vi "Compute Centroid.vi"(0 "Pixel0":bool, 1 "Image Width":u16, 4 "Image Height":u16, 5 "Input Valid":bool, 7 "Pixel5":bool, 8 "Pixel1":bool, 9 "Pixel6":bool, 10 "Pixel2":bool, 11 "Pixel7":bool, 12 "Pixel3":bool, 13 "Pixel8":bool, 14 "Pixel4":bool, 15 "Pixel9":bool) -> (20 "X":fxp<+,32,16>, 21 "Y":fxp<+,32,16>, 22 "Output valid":bool, 24 "Ymin":u16, 25 "Ymax":u16, 26 "Xmin":u16, 27 "Xmax":u16)   [LabVIEW 2014]
doc: "This VI computes the centroid of a binary image. It is intended to be run on an FPGA."
uses:
  <vilib>/rvi/FXPMathLib/FxpDiv/subVIs/nifxpmath_Div_SimConfig.ctl
  <vilib>/rvi/FXPMathLib/FxpDiv/simVIs/DllFxpDivTemp_sub.vi
  <vilib>/rvi/FXPMathLib/FxpDiv/XNode/nifxpmath_Div.xnode
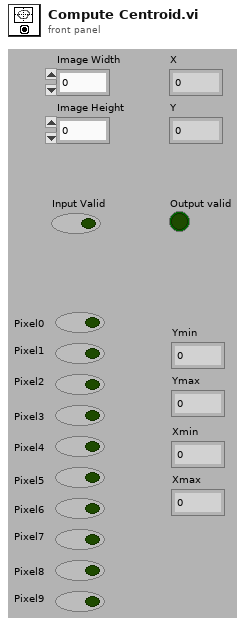
[diagram p1: front panel]
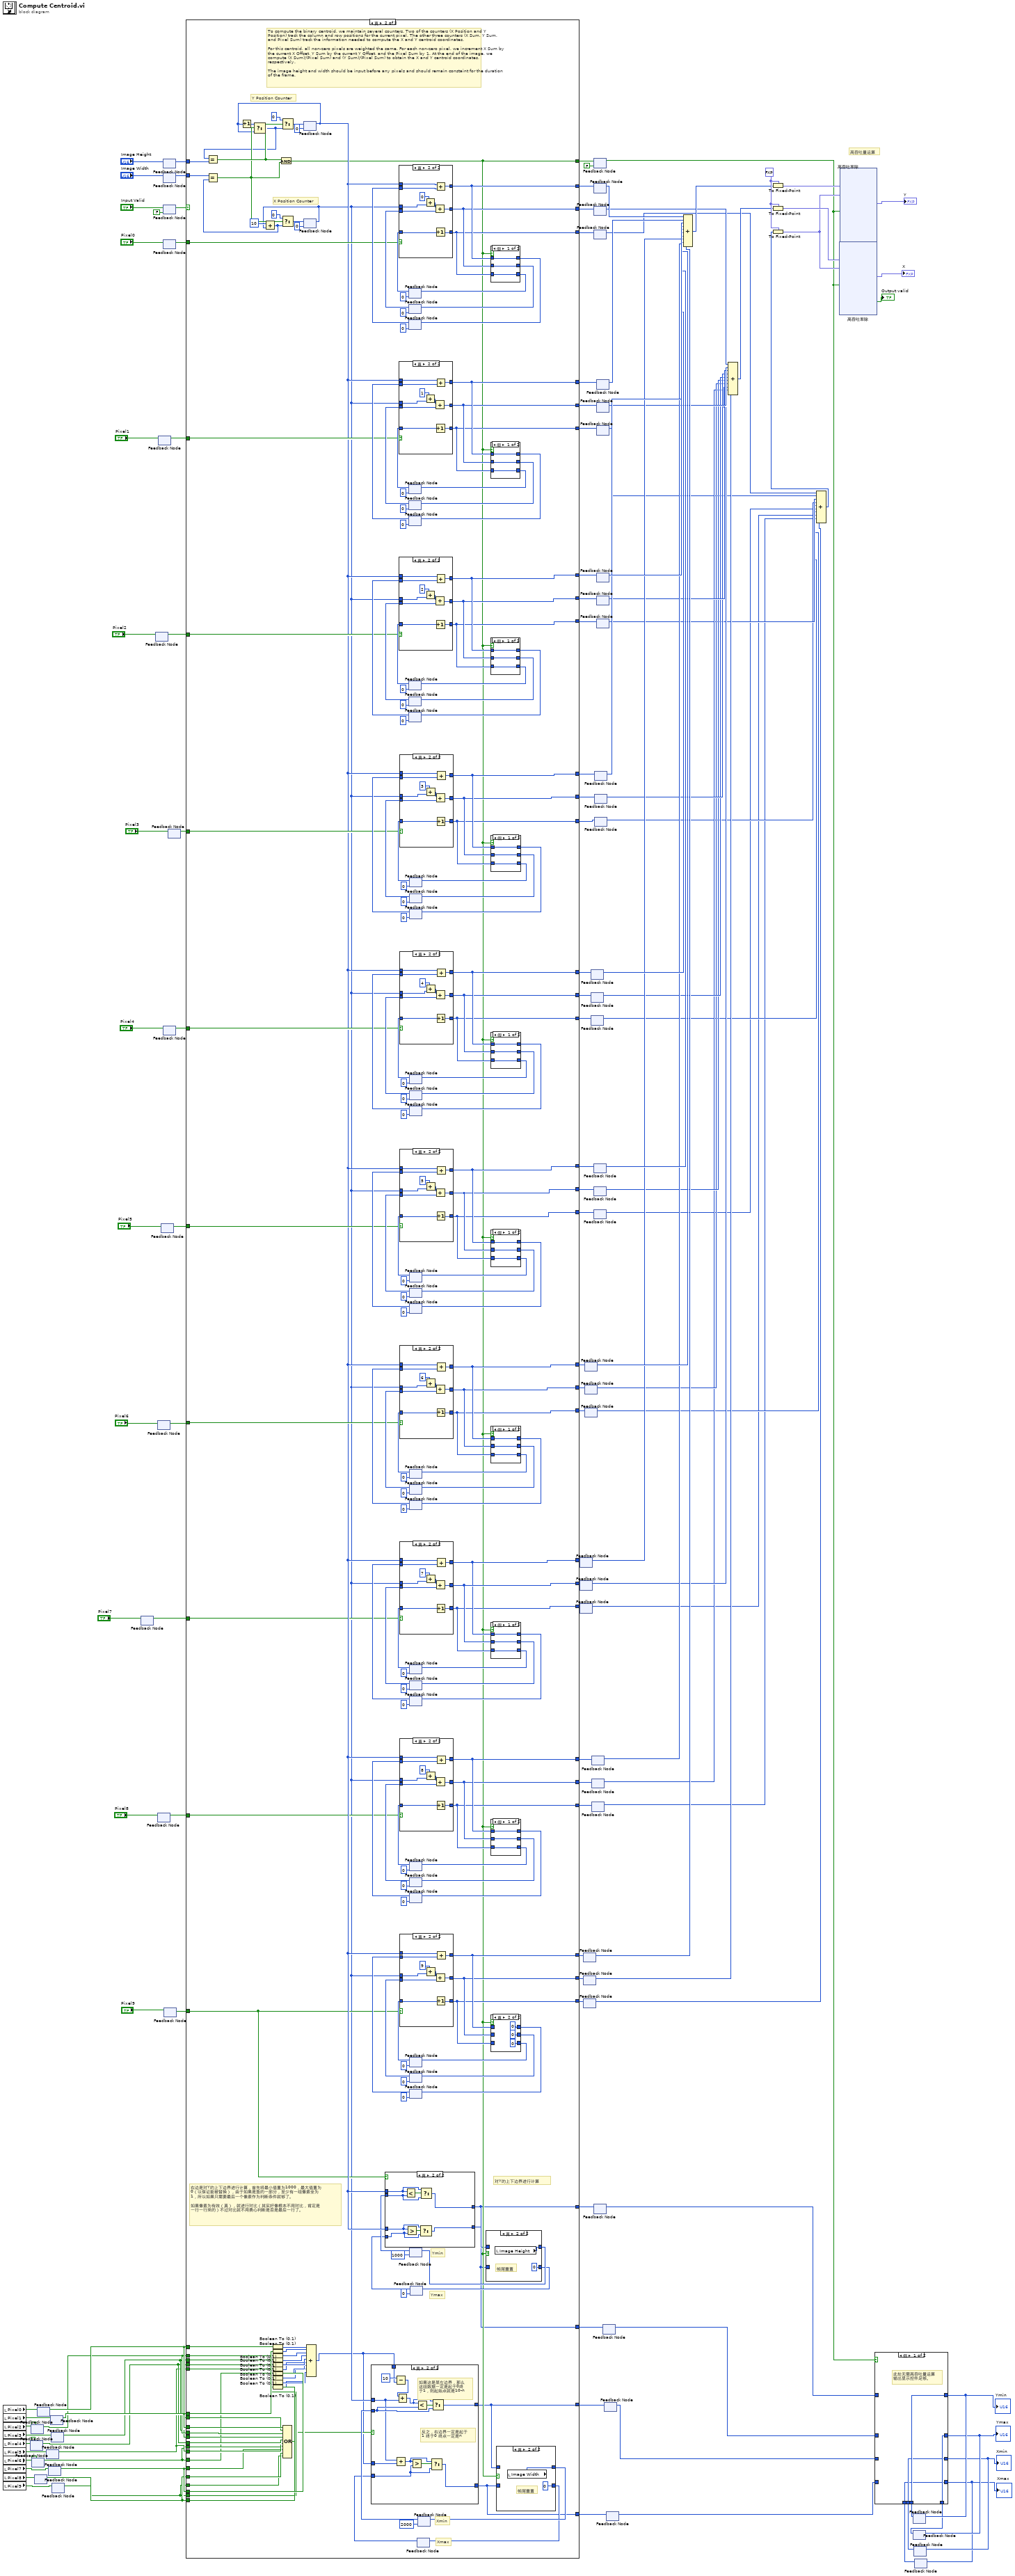
[diagram p0: block diagram]
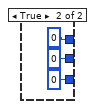
[diagram p10: hidden frame]
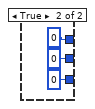
[diagram p12: hidden frame]
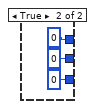
[diagram p14: hidden frame]
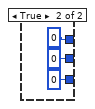
[diagram p16: hidden frame]
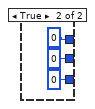
[diagram p18: hidden frame]
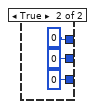
[diagram p20: hidden frame]
diagram:
  w125 = fxp<+,32,32> 0.0 ("fixed-point type")
  # "高吞吐量运算"
  n1 = local read "Pixel0"() -> (w37:bool)
  n2 = local read "Pixel1"() -> (w36:bool)
  n3 = local read "Pixel2"() -> (w35:bool)
  n4 = local read "Pixel3"() -> (w34:bool)
  n5 = local read "Pixel4"() -> (w33:bool)
  n6 = local read "Pixel5"() -> (w32:bool)
  n7 = local read "Pixel6"() -> (w31:bool)
  n8 = local read "Pixel7"() -> (w30:bool)
  n9 = local read "Pixel8"() -> (w29:bool)
  n10 = local read "Pixel9"() -> (w28:bool)
  n11 = feedback-in #1(w33) -> ()
  n12 = feedback #1() -> (w6:bool)  [unwired: 1 in]
  n13 = feedback-in #2(w35) -> ()
  n14 = feedback #2() -> (w8:bool)  [unwired: 1 in]
  n15 = feedback-in #3(w31) -> ()
  n16 = feedback #3() -> (w4:bool)  [unwired: 1 in]
  n17 = feedback-in #4(w29) -> ()
  n18 = feedback #4() -> (w2:bool)  [unwired: 1 in]
  n19 = feedback-in #5(w37) -> ()
  n20 = feedback #5() -> (w10:bool)  [unwired: 1 in]
  n21 = feedback-in #6(w32) -> ()
  n22 = feedback #6() -> (w5:bool)  [unwired: 1 in]
  n23 = feedback-in #7(w30) -> ()
  n24 = feedback #7() -> (w3:bool)  [unwired: 1 in]
  n25 = feedback-in #8(w36) -> ()
  n26 = feedback #8() -> (w9:bool)  [unwired: 1 in]
  n27 = feedback-in #9(w34) -> ()
  n28 = feedback #9() -> (w7:bool)  [unwired: 1 in]
  n29 = feedback-in #10(w28) -> ()
  n30 = feedback #10() -> (w1:bool)  [unwired: 1 in]
  n31 = feedback #11() -> (w75:bool)  [unwired: 1 in]
  n32 = feedback-in #11("Pixel7") -> ()
  n33 = feedback #12() -> (w109:bool)  [unwired: 1 in]
  n34 = feedback-in #12("Pixel2") -> ()
  n35 = feedback #13() -> (w73:bool)  [unwired: 1 in]
  n36 = feedback-in #13("Pixel8") -> ()
  n37 = feedback #14() -> (w77:bool)  [unwired: 1 in]
  n38 = feedback-in #14("Pixel6") -> ()
  n39 = feedback #15() -> (w114:bool)  [unwired: 1 in]
  n40 = feedback-in #15("Pixel1") -> ()
  n41 = feedback #16() -> (w79:bool)  [unwired: 1 in]
  n42 = feedback-in #16("Pixel5") -> ()
  n43 = feedback #17() -> (w99:bool)  [unwired: 1 in]
  n44 = feedback-in #17("Pixel4") -> ()
  n45 = feedback #18() -> (w131:u16)  [unwired: 1 in]
  n46 = feedback-in #18("Image Height") -> ()
  n47 = feedback #19() -> (w130:u16)  [unwired: 1 in]
  n48 = feedback-in #19("Image Width") -> ()
  n49 = feedback #20(FALSE ("Input Valid")) -> (w132:bool)
  n50 = feedback-in #20("Input Valid") -> ()
  n51 = feedback #21() -> (w129:bool)  [unwired: 1 in]
  n52 = feedback-in #21("Pixel0") -> ()
  n53 = feedback #22() -> (w71:bool)  [unwired: 1 in]
  n54 = feedback-in #22("Pixel9") -> ()
  n55 = feedback #23() -> (w104:bool)  [unwired: 1 in]
  n56 = feedback-in #23("Pixel3") -> ()
  n57 = case shown="真" w132 {
    tunnel: [_ w145] -> w120
    tunnel: w131 -> [_ w314]
    tunnel: w130 -> [_ w309]
    tunnel: w129 -> [_ w315]
    tunnel: [_ w307] -> w117
    tunnel: [_ w306] -> w118
    tunnel: [_ w305] -> w119
    tunnel: w114 -> [_ w295]
    tunnel: [_ w294] -> w113
    tunnel: [_ w293] -> w112
    tunnel: [_ w292] -> w111
    tunnel: w109 -> [_ w219]
    tunnel: [_ w218] -> w108
    tunnel: [_ w217] -> w107
    tunnel: [_ w216] -> w106
    tunnel: w104 -> [_ w215]
    tunnel: [_ w214] -> w103
    tunnel: [_ w213] -> w102
    tunnel: [_ w212] -> w101
    tunnel: w99 -> [_ w211]
    tunnel: [_ w210] -> w98
    tunnel: [_ w209] -> w97
    tunnel: [_ w208] -> w96
    tunnel: [_ w207] -> w95
    tunnel: [_ w206] -> w94
    tunnel: [_ w205] -> w93
    tunnel: [_ w204] -> w92
    tunnel: [_ w203] -> w91
    tunnel: [_ w202] -> w90
    tunnel: [_ w201] -> w89
    tunnel: [_ w200] -> w88
    tunnel: [_ w199] -> w87
    tunnel: [_ w198] -> w86
    tunnel: [_ w197] -> w85
    tunnel: [_ w196] -> w84
    tunnel: [_ w195] -> w83
    tunnel: [_ w194] -> w82
    tunnel: [_ w193] -> w81
    tunnel: w79 -> [_ w192]
    tunnel: w77 -> [_ w191]
    tunnel: w75 -> [_ w180]
    tunnel: w73 -> [_ w181]
    tunnel: w71 -> [_ w182]
    tunnel: w10 -> [_ w179]
    tunnel: w9 -> [_ w178]
    tunnel: w8 -> [_ w177]
    tunnel: w7 -> [_ w176]
    tunnel: w6 -> [_ w175]
    tunnel: w5 -> [_ w174]
    tunnel: w4 -> [_ w173]
    tunnel: w3 -> [_ w172]
    tunnel: w2 -> [_ w171]
    tunnel: w1 -> [_ w170]
    tunnel: w10 -> [_ w169]
    tunnel: w9 -> [_ w168]
    tunnel: w8 -> [_ w167]
    tunnel: w7 -> [_ w166]
    tunnel: w6 -> [_ w165]
    tunnel: w5 -> [_ w164]
    tunnel: w4 -> [_ w163]
    tunnel: w3 -> [_ w162]
    tunnel: w2 -> [_ w161]
    tunnel: w1 -> [_ w160]
    tunnel: [_ w142] -> w26
    tunnel: [_ w141] -> w24
    tunnel: [_ w140] -> w23
    tunnel: [_ w139] -> w22
    frame False {
      # "If the input is not valid, then do not update the accumulators."
    }
    frame True {
      # "右边是对Y的上下边界进行计算，首先将最小值置为1000，最大值置为\n0（以保证能被替换），由于如果是鱼的一部分，至少有一组像素全为\n1，所以如果只需要最后一个像素作为判断条件就够了。\n\n如果像素为有效（真），就进行对比（其实好像根本不用对比，肯定是\n一行一行来的）不过对比就不用费心判断是否是最后一行了。"
      # "Xmax"
      # "Xmin"
      # "对Y的上下边界进行计算"
      # "Ymax"
      # "Ymin"
      # "To compute the binary centroid, we maintain several counters. Two of the counters (X Position and Y Position) track the column and row positions for the current pixel. The other three counters (X Sum, Y Sum, and Pixel Sum) track the information needed to compute the X and Y centroid coordinates.\n\nFor this centroid, all non-zero pixels are weighted the same. For each non-zero pixel, we increment X Sum by the current X Offset, Y Sum by the current Y Offset, and the Pixel Sum by 1. At the end of the image, we compute (X Sum)/(Pixel Sum) and (Y Sum)/(Pixel Sum) to obtain the X and Y centroid coordinates, respectively.\n\nThe image height and width should be input before any pixels and should remain constaint for the duration of the frame."
      # "X Position Counter"
      # "Y Position Counter"
      n58 = Boolean To (0,1)(Boolean=w169) -> (0, 1=w159:i16)
      n59 = Boolean To (0,1)(Boolean=w168) -> (0, 1=w158:i16)
      n60 = Boolean To (0,1)(Boolean=w167) -> (0, 1=w157:i16)
      n61 = Boolean To (0,1)(Boolean=w166) -> (0, 1=w156:i16)
      n62 = Boolean To (0,1)(Boolean=w165) -> (0, 1=w155:i16)
      n63 = Boolean To (0,1)(Boolean=w164) -> (0, 1=w154:i16)
      n64 = Boolean To (0,1)(Boolean=w163) -> (0, 1=w153:i16)
      n65 = Boolean To (0,1)(Boolean=w162) -> (0, 1=w152:i16)
      n66 = Boolean To (0,1)(Boolean=w161) -> (0, 1=w151:i16)
      n67 = Boolean To (0,1)(Boolean=w160) -> (0, 1=w150:i16)
      n68 = Compound Arithmetic op=OR(w179, w178, w177, w176, w175, w174, w173, w172, w171, w170) -> (w138:bool)
      n69 = feedback #24(u16 0 ("t")) -> (w187:u16)
      n70 = Increment(x=w187) -> (x+1=w312:u16)
      n71 = feedback #25(u16 0 ("t")) -> (w149:u16)
      n72 = Add(x=u16 10, y=w149) -> (x+y=w308:u16)
      n73 = Equal?(x=w309, y=w308) -> (x = y?=w323:bool)
      n74 = Select(t=w312, s=w323, f=w187) -> (s? t:f=w311:u16)
      n75 = Equal?(x=w311, y=w314) -> (x = y?=w326:bool)
      n76 = And(x=w326, y=w323) -> (x .and. y?=w145:bool)
      n77 = Select(t=u16 0, s=w326, f=w311) -> (s? t:f=w317:u16)
      n78 = Select(t=u16 0, s=w323, f=w308) -> (s? t:f=w319:u16)
      n79 = feedback-in #24(w317) -> ()
      n80 = feedback-in #25(w319) -> ()
      n81 = Compound Arithmetic op=ADD(w159, w158, w157, w156, w155, w154, w153, w152, w151, w150) -> (w137:i16)
      n82 = feedback #26(u32 0 ("Pixel 0")) -> (w321:u32)
      n83 = feedback #27(u32 0 ("Pixel 0")) -> (w330:u32)
      n84 = feedback #28(u32 0 ("Pixel 0")) -> (w329:u32)
      n85 = case shown="真" w315 {
        tunnel: [w543 w553] -> w306
        tunnel: w330 -> [w543 w552]
        tunnel: w329 -> [w542 w551]
        tunnel: [w542 w550] -> w307
        tunnel: w149 -> [_ w544]
        tunnel: w187 -> [_ w549]
        tunnel: [w541 w548] -> w305
        tunnel: w321 -> [w541 w547]
        frame False {
        }
        frame True {
          n86 = Add(x=u16 0, y=w544) -> (x+y=w545:u16)
          n87 = Add(x=w545, y=w552) -> (x+y=w553:u32)
          n88 = Increment(x=w547) -> (x+1=w548:u32)
          n89 = Add(x=w549, y=w551) -> (x+y=w550:u32)
        }
      }
      n90 = feedback #29(u32 0 ("Pixel 0")) -> (w297:u32)
      n91 = feedback #30(u32 0 ("Pixel 0")) -> (w304:u32)
      n92 = feedback #31(u32 0 ("Pixel 0")) -> (w303:u32)
      n93 = case shown="真" w295 {
        tunnel: [w524 w534] -> w293
        tunnel: w304 -> [w524 w533]
        tunnel: w303 -> [w523 w532]
        tunnel: [w523 w531] -> w294
        tunnel: w149 -> [_ w525]
        tunnel: w187 -> [_ w530]
        tunnel: [w522 w529] -> w292
        tunnel: w297 -> [w522 w528]
        frame False {
        }
        frame True {
          n94 = Add(x=u16 1, y=w525) -> (x+y=w526:u16)
          n95 = Add(x=w526, y=w533) -> (x+y=w534:u32)
          n96 = Increment(x=w528) -> (x+1=w529:u32)
          n97 = Add(x=w530, y=w532) -> (x+y=w531:u32)
        }
      }
      n98 = feedback #32(u32 0 ("Pixel 0")) -> (w284:u32)
      n99 = feedback #33(u32 0 ("Pixel 0")) -> (w291:u32)
      n100 = feedback #34(u32 0 ("Pixel 0")) -> (w290:u32)
      n101 = case shown="真" w219 {
        tunnel: [w505 w515] -> w217
        tunnel: w291 -> [w505 w514]
        tunnel: w290 -> [w504 w513]
        tunnel: [w504 w512] -> w218
        tunnel: w149 -> [_ w506]
        tunnel: w187 -> [_ w511]
        tunnel: [w503 w510] -> w216
        tunnel: w284 -> [w503 w509]
        frame False {
        }
        frame True {
          n102 = Add(x=u16 2, y=w506) -> (x+y=w507:u16)
          n103 = Add(x=w507, y=w514) -> (x+y=w515:u32)
          n104 = Increment(x=w509) -> (x+1=w510:u32)
          n105 = Add(x=w511, y=w513) -> (x+y=w512:u32)
        }
      }
      n106 = feedback #35(u32 0 ("Pixel 0")) -> (w275:u32)
      n107 = feedback #36(u32 0 ("Pixel 0")) -> (w282:u32)
      n108 = feedback #37(u32 0 ("Pixel 0")) -> (w281:u32)
      n109 = case shown="真" w215 {
        tunnel: [w486 w496] -> w213
        tunnel: w282 -> [w486 w495]
        tunnel: w281 -> [w485 w494]
        tunnel: [w485 w493] -> w214
        tunnel: w149 -> [_ w487]
        tunnel: w187 -> [_ w492]
        tunnel: [w484 w491] -> w212
        tunnel: w275 -> [w484 w490]
        frame False {
        }
        frame True {
          n110 = Add(x=u16 3, y=w487) -> (x+y=w488:u16)
          n111 = Add(x=w488, y=w495) -> (x+y=w496:u32)
          n112 = Increment(x=w490) -> (x+1=w491:u32)
          n113 = Add(x=w492, y=w494) -> (x+y=w493:u32)
        }
      }
      n114 = feedback #38(u32 0 ("Pixel 0")) -> (w266:u32)
      n115 = feedback #39(u32 0 ("Pixel 0")) -> (w273:u32)
      n116 = feedback #40(u32 0 ("Pixel 0")) -> (w272:u32)
      n117 = case shown="真" w211 {
        tunnel: [w467 w477] -> w209
        tunnel: w273 -> [w467 w476]
        tunnel: w272 -> [w466 w475]
        tunnel: [w466 w474] -> w210
        tunnel: w149 -> [_ w468]
        tunnel: w187 -> [_ w473]
        tunnel: [w465 w472] -> w208
        tunnel: w266 -> [w465 w471]
        frame False {
        }
        frame True {
          n118 = Add(x=u16 4, y=w468) -> (x+y=w469:u16)
          n119 = Add(x=w469, y=w476) -> (x+y=w477:u32)
          n120 = Increment(x=w471) -> (x+1=w472:u32)
          n121 = Add(x=w473, y=w475) -> (x+y=w474:u32)
        }
      }
      n122 = feedback #41(u32 0 ("Pixel 0")) -> (w257:u32)
      n123 = feedback #42(u32 0 ("Pixel 0")) -> (w264:u32)
      n124 = feedback #43(u32 0 ("Pixel 0")) -> (w263:u32)
      n125 = case shown="真" w192 {
        tunnel: [w448 w458] -> w206
        tunnel: w264 -> [w448 w457]
        tunnel: w263 -> [w447 w456]
        tunnel: [w447 w455] -> w207
        tunnel: w149 -> [_ w449]
        tunnel: w187 -> [_ w454]
        tunnel: [w446 w453] -> w205
        tunnel: w257 -> [w446 w452]
        frame False {
        }
        frame True {
          n126 = Add(x=u16 5, y=w449) -> (x+y=w450:u16)
          n127 = Add(x=w450, y=w457) -> (x+y=w458:u32)
          n128 = Increment(x=w452) -> (x+1=w453:u32)
          n129 = Add(x=w454, y=w456) -> (x+y=w455:u32)
        }
      }
      n130 = feedback #44(u32 0 ("Pixel 0")) -> (w248:u32)
      n131 = feedback #45(u32 0 ("Pixel 0")) -> (w255:u32)
      n132 = feedback #46(u32 0 ("Pixel 0")) -> (w254:u32)
      n133 = case shown="真" w191 {
        tunnel: [w429 w439] -> w203
        tunnel: w255 -> [w429 w438]
        tunnel: w254 -> [w428 w437]
        tunnel: [w428 w436] -> w204
        tunnel: w149 -> [_ w430]
        tunnel: w187 -> [_ w435]
        tunnel: [w427 w434] -> w202
        tunnel: w248 -> [w427 w433]
        frame False {
        }
        frame True {
          n134 = Add(x=u16 6, y=w430) -> (x+y=w431:u16)
          n135 = Add(x=w431, y=w438) -> (x+y=w439:u32)
          n136 = Increment(x=w433) -> (x+1=w434:u32)
          n137 = Add(x=w435, y=w437) -> (x+y=w436:u32)
        }
      }
      n138 = feedback #47(u32 0 ("Pixel 0")) -> (w239:u32)
      n139 = feedback #48(u32 0 ("Pixel 0")) -> (w246:u32)
      n140 = feedback #49(u32 0 ("Pixel 0")) -> (w245:u32)
      n141 = case shown="真" w180 {
        tunnel: [w410 w420] -> w201
        tunnel: w246 -> [w410 w419]
        tunnel: w245 -> [w409 w418]
        tunnel: [w409 w417] -> w200
        tunnel: w149 -> [_ w411]
        tunnel: w187 -> [_ w416]
        tunnel: [w408 w415] -> w199
        tunnel: w239 -> [w408 w414]
        frame False {
        }
        frame True {
          n142 = Add(x=u16 7, y=w411) -> (x+y=w412:u16)
          n143 = Add(x=w412, y=w419) -> (x+y=w420:u32)
          n144 = Increment(x=w414) -> (x+1=w415:u32)
          n145 = Add(x=w416, y=w418) -> (x+y=w417:u32)
        }
      }
      n146 = feedback #50(u32 0 ("Pixel 0")) -> (w230:u32)
      n147 = feedback #51(u32 0 ("Pixel 0")) -> (w237:u32)
      n148 = feedback #52(u32 0 ("Pixel 0")) -> (w236:u32)
      n149 = case shown="真" w181 {
        tunnel: [w391 w401] -> w197
        tunnel: w237 -> [w391 w400]
        tunnel: w236 -> [w390 w399]
        tunnel: [w390 w398] -> w198
        tunnel: w149 -> [_ w392]
        tunnel: w187 -> [_ w397]
        tunnel: [w389 w396] -> w196
        tunnel: w230 -> [w389 w395]
        frame False {
        }
        frame True {
          n150 = Add(x=u16 8, y=w392) -> (x+y=w393:u16)
          n151 = Add(x=w393, y=w400) -> (x+y=w401:u32)
          n152 = Increment(x=w395) -> (x+1=w396:u32)
          n153 = Add(x=w397, y=w399) -> (x+y=w398:u32)
        }
      }
      n154 = feedback #53(u32 0 ("Pixel 0")) -> (w221:u32)
      n155 = feedback #54(u32 0 ("Pixel 0")) -> (w228:u32)
      n156 = feedback #55(u32 0 ("Pixel 0")) -> (w227:u32)
      n157 = case shown="真" w182 {
        tunnel: [w372 w382] -> w194
        tunnel: w228 -> [w372 w381]
        tunnel: w227 -> [w371 w380]
        tunnel: [w371 w379] -> w195
        tunnel: w149 -> [_ w373]
        tunnel: w187 -> [_ w378]
        tunnel: [w370 w377] -> w193
        tunnel: w221 -> [w370 w376]
        frame False {
        }
        frame True {
          n158 = Add(x=u16 9, y=w373) -> (x+y=w374:u16)
          n159 = Add(x=w374, y=w381) -> (x+y=w382:u32)
          n160 = Increment(x=w376) -> (x+1=w377:u32)
          n161 = Add(x=w378, y=w380) -> (x+y=w379:u32)
        }
      }
      n162 = feedback #56(u16 1000 ("Image Width")) -> (w186:u16)
      n163 = feedback #57(u16 0 ("t")) -> (w184:u16)
      n164 = case shown="真" w182 {
        tunnel: w187 -> [_ w362]
        tunnel: w186 -> [w355 w361]
        tunnel: [w355 w360] -> w142
        tunnel: w187 -> [_ w358]
        tunnel: [w354 w357] -> w141
        tunnel: w184 -> [w354 w356]
        frame False {
        }
        frame True {
          n165 = Less?(x=w362, y=w361) -> (x < y?=w363:bool)
          n166 = Greater?(x=w358, y=w356) -> (0:w359:bool)
          n167 = Select(t=w358, s=w359, f=w356) -> (s? t:f=w357:u16)
          n168 = Select(t=w362, s=w363, f=w361) -> (s? t:f=w360:u16)
        }
      }
      n169 = feedback #58() -> (w144:u16)  [unwired: 1 in]
      n170 = feedback #59(u16 2000) -> (w148:u16)
      n171 = case shown="真" w138 {
        tunnel: w137 -> [_ w348]
        tunnel: w149 -> [_ w342]
        tunnel: w148 -> [w336 w345]
        tunnel: [w336 w343] -> w140
        tunnel: w137 -> [_ w341]
        tunnel: w144 -> [w335 w338]
        tunnel: [w335 w337] -> w139
        frame False {
        }
        frame True {
          # "反之，右边界一定是起于\n1 终于0 终点一定是n"
          # "如果这是某左边界，那么\n这组数据一定是起于0终\n于1，则起始点就是10-n"
          n172 = Subtract(x=i16 10, y=w348) -> (x-y=w347:i16)
          n173 = Add(x=w342, y=w341) -> (x+y=w339:u16)
          n174 = Add(x=w347, y=w342) -> (x+y=w344:u16)
          n175 = Greater?(x=w339, y=w338) -> (0:w340:bool)
          n176 = Less?(x=w344, y=w345) -> (x < y?=w346:bool)
          n177 = Select(t=w339, s=w340, f=w338) -> (s? t:f=w337:u16)
          n178 = Select(t=w344, s=w346, f=w345) -> (s? t:f=w343:u16)
        }
      }
      n179 = case shown="真" w145 {
        tunnel: [w351 w353] -> w189
        tunnel: w142 -> [w351 _]
        tunnel: w141 -> [w350 _]
        tunnel: [w350 u16 0 ("t")] -> w185
        frame False {
        }
        frame True {
          # "帧尾重置"
          n180 = local read "Image Height"() -> (w353:u16)
        }
      }
      n181 = feedback-in #56(w189) -> ()
      n182 = feedback-in #57(w185) -> ()
      n183 = case shown="假" w145 {
        tunnel: w306 -> [w536 _]
        tunnel: [w536 u32 0 ("Pixel 0")] -> w325
        tunnel: w307 -> [w537 _]
        tunnel: [w537 u32 0 ("Pixel 0")] -> w324
        tunnel: w305 -> [w535 _]
        tunnel: [w535 u32 0 ("Pixel 0")] -> w322
        frame False {
        }
        frame True {
        }
      }
      n184 = feedback-in #26(w322) -> ()
      n185 = feedback-in #27(w325) -> ()
      n186 = feedback-in #28(w324) -> ()
      n187 = case shown="假" w145 {
        tunnel: w293 -> [w517 _]
        tunnel: [w517 u32 0 ("Pixel 0")] -> w300
        tunnel: w294 -> [w518 _]
        tunnel: [w518 u32 0 ("Pixel 0")] -> w299
        tunnel: w292 -> [w516 _]
        tunnel: [w516 u32 0 ("Pixel 0")] -> w298
        frame False {
        }
        frame True {
        }
      }
      n188 = feedback-in #29(w298) -> ()
      n189 = feedback-in #30(w300) -> ()
      n190 = feedback-in #31(w299) -> ()
      n191 = case shown="假" w145 {
        tunnel: w217 -> [w498 _]
        tunnel: [w498 u32 0 ("Pixel 0")] -> w287
        tunnel: w218 -> [w499 _]
        tunnel: [w499 u32 0 ("Pixel 0")] -> w286
        tunnel: w216 -> [w497 _]
        tunnel: [w497 u32 0 ("Pixel 0")] -> w285
        frame False {
        }
        frame True {
        }
      }
      n192 = feedback-in #32(w285) -> ()
      n193 = feedback-in #33(w287) -> ()
      n194 = feedback-in #34(w286) -> ()
      n195 = case shown="假" w145 {
        tunnel: w213 -> [w479 _]
        tunnel: [w479 u32 0 ("Pixel 0")] -> w278
        tunnel: w214 -> [w480 _]
        tunnel: [w480 u32 0 ("Pixel 0")] -> w277
        tunnel: w212 -> [w478 _]
        tunnel: [w478 u32 0 ("Pixel 0")] -> w276
        frame False {
        }
        frame True {
        }
      }
      n196 = feedback-in #35(w276) -> ()
      n197 = feedback-in #36(w278) -> ()
      n198 = feedback-in #37(w277) -> ()
      n199 = case shown="假" w145 {
        tunnel: w209 -> [w460 _]
        tunnel: [w460 u32 0 ("Pixel 0")] -> w269
        tunnel: w210 -> [w461 _]
        tunnel: [w461 u32 0 ("Pixel 0")] -> w268
        tunnel: w208 -> [w459 _]
        tunnel: [w459 u32 0 ("Pixel 0")] -> w267
        frame False {
        }
        frame True {
        }
      }
      n200 = feedback-in #38(w267) -> ()
      n201 = feedback-in #39(w269) -> ()
      n202 = feedback-in #40(w268) -> ()
      n203 = case shown="假" w145 {
        tunnel: w206 -> [w441 _]
        tunnel: [w441 u32 0 ("Pixel 0")] -> w260
        tunnel: w207 -> [w442 _]
        tunnel: [w442 u32 0 ("Pixel 0")] -> w259
        tunnel: w205 -> [w440 _]
        tunnel: [w440 u32 0 ("Pixel 0")] -> w258
        frame False {
        }
        frame True {
        }
      }
      n204 = feedback-in #41(w258) -> ()
      n205 = feedback-in #42(w260) -> ()
      n206 = feedback-in #43(w259) -> ()
      n207 = case shown="假" w145 {
        tunnel: w203 -> [w422 _]
        tunnel: [w422 u32 0 ("Pixel 0")] -> w251
        tunnel: w204 -> [w423 _]
        tunnel: [w423 u32 0 ("Pixel 0")] -> w250
        tunnel: w202 -> [w421 _]
        tunnel: [w421 u32 0 ("Pixel 0")] -> w249
        frame False {
        }
        frame True {
        }
      }
      n208 = feedback-in #44(w249) -> ()
      n209 = feedback-in #45(w251) -> ()
      n210 = feedback-in #46(w250) -> ()
      n211 = case shown="假" w145 {
        tunnel: w201 -> [w403 _]
        tunnel: [w403 u32 0 ("Pixel 0")] -> w242
        tunnel: w200 -> [w404 _]
        tunnel: [w404 u32 0 ("Pixel 0")] -> w241
        tunnel: w199 -> [w402 _]
        tunnel: [w402 u32 0 ("Pixel 0")] -> w240
        frame False {
        }
        frame True {
        }
      }
      n212 = feedback-in #47(w240) -> ()
      n213 = feedback-in #48(w242) -> ()
      n214 = feedback-in #49(w241) -> ()
      n215 = case shown="假" w145 {
        tunnel: w197 -> [w384 _]
        tunnel: [w384 u32 0 ("Pixel 0")] -> w233
        tunnel: w198 -> [w385 _]
        tunnel: [w385 u32 0 ("Pixel 0")] -> w232
        tunnel: w196 -> [w383 _]
        tunnel: [w383 u32 0 ("Pixel 0")] -> w231
        frame False {
        }
        frame True {
        }
      }
      n216 = feedback-in #50(w231) -> ()
      n217 = feedback-in #51(w233) -> ()
      n218 = feedback-in #52(w232) -> ()
      n219 = case shown="真" w145 {
        tunnel: w194 -> [w365 _]
        tunnel: [w365 u32 0 ("Pixel 0")] -> w224
        tunnel: w195 -> [w366 _]
        tunnel: [w366 u32 0 ("Pixel 0")] -> w223
        tunnel: w193 -> [w364 _]
        tunnel: [w364 u32 0 ("Pixel 0")] -> w222
        frame False {
        }
        frame True {
        }
      }
      n220 = feedback-in #53(w222) -> ()
      n221 = feedback-in #54(w224) -> ()
      n222 = feedback-in #55(w223) -> ()
      n223 = case shown="真" w145 {
        tunnel: [w332 w334] -> w147
        tunnel: w140 -> [w332 _]
        tunnel: [w331 u16 0] -> w143
        tunnel: w139 -> [w331 _]
        frame False {
        }
        frame True {
          # "帧尾重置"
          n224 = local read "Image Width"() -> (w334:u16)
        }
      }
      n225 = feedback-in #58(w143) -> ()
      n226 = feedback-in #59(w147) -> ()
    }
  }
  n227 = feedback #60() -> (w63:u32)  [unwired: 1 in]
  n228 = feedback-in #60(w88) -> ()
  n229 = feedback #61() -> (w52:u32)  [unwired: 1 in]
  n230 = feedback-in #61(w89) -> ()
  n231 = feedback #62() -> (w41:u32)  [unwired: 1 in]
  n232 = feedback-in #62(w87) -> ()
  n233 = feedback #63() -> (w61:u32)  [unwired: 1 in]
  n234 = feedback-in #63(w83) -> ()
  n235 = feedback #64() -> (w50:u32)  [unwired: 1 in]
  n236 = feedback-in #64(w82) -> ()
  n237 = feedback #65() -> (w39:u32)  [unwired: 1 in]
  n238 = feedback-in #65(w81) -> ()
  n239 = feedback #66() -> (w64:u32)  [unwired: 1 in]
  n240 = feedback-in #66(w92) -> ()
  n241 = feedback #67() -> (w53:u32)  [unwired: 1 in]
  n242 = feedback-in #67(w91) -> ()
  n243 = feedback #68() -> (w42:u32)  [unwired: 1 in]
  n244 = feedback-in #68(w90) -> ()
  n245 = feedback #69() -> (w66:u32)  [unwired: 1 in]
  n246 = feedback-in #69(w98) -> ()
  n247 = feedback #70() -> (w55:u32)  [unwired: 1 in]
  n248 = feedback-in #70(w97) -> ()
  n249 = feedback #71() -> (w44:u32)  [unwired: 1 in]
  n250 = feedback-in #71(w96) -> ()
  n251 = feedback #72() -> (w62:u32)  [unwired: 1 in]
  n252 = feedback-in #72(w86) -> ()
  n253 = feedback #73() -> (w51:u32)  [unwired: 1 in]
  n254 = feedback-in #73(w85) -> ()
  n255 = feedback #74() -> (w40:u32)  [unwired: 1 in]
  n256 = feedback-in #74(w84) -> ()
  n257 = feedback-in #75(w120) -> ()
  n258 = feedback #75(FALSE) -> (w27:bool)
  n259 = feedback #76() -> (w70:u32)  [unwired: 1 in]
  n260 = feedback-in #76(w117) -> ()
  n261 = feedback #77() -> (w59:u32)  [unwired: 1 in]
  n262 = feedback-in #77(w118) -> ()
  n263 = feedback #78() -> (w48:u32)  [unwired: 1 in]
  n264 = feedback-in #78(w119) -> ()
  n265 = feedback-in #79(w26) -> ()
  n266 = feedback #79() -> (w14:u16)  [unwired: 1 in]
  n267 = feedback #80() -> (w65:u32)  [unwired: 1 in]
  n268 = feedback-in #80(w95) -> ()
  n269 = feedback #81() -> (w54:u32)  [unwired: 1 in]
  n270 = feedback-in #81(w94) -> ()
  n271 = feedback #82() -> (w43:u32)  [unwired: 1 in]
  n272 = feedback-in #82(w93) -> ()
  n273 = feedback #83() -> (w67:u32)  [unwired: 1 in]
  n274 = feedback-in #83(w103) -> ()
  n275 = feedback #84() -> (w56:u32)  [unwired: 1 in]
  n276 = feedback-in #84(w102) -> ()
  n277 = feedback #85() -> (w45:u32)  [unwired: 1 in]
  n278 = feedback-in #85(w101) -> ()
  n279 = feedback #86() -> (w69:u32)  [unwired: 1 in]
  n280 = feedback-in #86(w113) -> ()
  n281 = feedback #87() -> (w58:u32)  [unwired: 1 in]
  n282 = feedback-in #87(w112) -> ()
  n283 = feedback #88() -> (w47:u32)  [unwired: 1 in]
  n284 = feedback-in #88(w111) -> ()
  n285 = feedback #89() -> (w68:u32)  [unwired: 1 in]
  n286 = feedback-in #89(w108) -> ()
  n287 = feedback #90() -> (w57:u32)  [unwired: 1 in]
  n288 = feedback-in #90(w107) -> ()
  n289 = feedback #91() -> (w46:u32)  [unwired: 1 in]
  n290 = feedback-in #91(w106) -> ()
  n291 = feedback-in #92(w24) -> ()
  n292 = feedback #92() -> (w13:u16)  [unwired: 1 in]
  n293 = feedback-in #93(w23) -> ()
  n294 = feedback #93() -> (w12:u16)  [unwired: 1 in]
  n295 = feedback-in #94(w22) -> ()
  n296 = feedback #94() -> (w11:u16)  [unwired: 1 in]
  n297 = Compound Arithmetic op=ADD(w70, w69, w68, w67, w66, w65, w64, w63, w62, w61) -> (w60:u32)
  n298 = Compound Arithmetic op=ADD(w59, w58, w57, w56, w55, w54, w53, w52, w51, w50) -> (w49:u32)
  n299 = To Fixed-Point(fixed-point type=w125, number=w60) -> (fixed-point=w124:fxp<+,32,32>)
  n300 = To Fixed-Point(fixed-point type=w125, number=w49) -> (fixed-point=w123:fxp<+,32,32>)
  n301 = Compound Arithmetic op=ADD(w48, w47, w46, w45, w44, w43, w42, w41, w40, w39) -> (w38:u32)
  n302 = To Fixed-Point(fixed-point type=w125, number=w38) -> (fixed-point=w122:fxp<+,32,32>)
  n303 = xnode "高吞吐率除"("x"=w123, "y"=w122, "输入有效"=w27) -> ("x/y"=→"X":fxp<+,32,16>, "输出有效"=→"Output valid":bool)  [unwired: 1 in, 1 out]
  n304 = xnode "高吞吐率除"("x"=w124, "y"=w122, "输入有效"=w27) -> ("x/y"=→"Y":fxp<+,32,16>)  [unwired: 1 in, 2 out]
  n305 = feedback #95() -> (w18:u16)  [unwired: 1 in]
  n306 = feedback #96() -> (w17:u16)  [unwired: 1 in]
  n307 = feedback #97() -> (w16:u16)  [unwired: 1 in]
  n308 = feedback #98() -> (w15:u16)  [unwired: 1 in]
  n309 = case shown="假" w27 {
    tunnel: [w557 w561] -> w25
    tunnel: w14 -> [_ w561]
    tunnel: [w556 w560] -> w21
    tunnel: w13 -> [_ w560]
    tunnel: [w555 w559] -> w20
    tunnel: w12 -> [_ w559]
    tunnel: [w554 w558] -> w19
    tunnel: w11 -> [_ w558]
    tunnel: w18 -> [w557 _]
    tunnel: w17 -> [w556 _]
    tunnel: w16 -> [w555 _]
    tunnel: w15 -> [w554 _]
    frame False {
      # "此处无需高吞吐量运算\n输出显示控件足够。"
    }
    frame True {
    }
  }
  "Ymin" <- w25
  "Ymax" <- w21
  "Xmin" <- w20
  "Xmax" <- w19
  n310 = feedback-in #95(w25) -> ()
  n311 = feedback-in #96(w21) -> ()
  n312 = feedback-in #97(w20) -> ()
  n313 = feedback-in #98(w19) -> ()
